vi "small_RT Main.vi"() -> ()   [LabVIEW 2018]
doc: "Demonstrates the use of the Network Streams functions to receive LED status from the host computer."
uses:
  <vilib>/myRIO/Instrument Drivers/Onboard IO/PWM/typedefs/PWM Reference.ctl
  <vilib>/myRIO/Common/Instrument Driver Framework/Utilities/typedefs/myRIO Generic Hardware Reference.ctl
  <vilib>/myRIO/Common/Instrument Driver Framework/Utilities/typedefs/Hardware Version Enum.ctl
  <vilib>/myRIO/Common/Instrument Driver Framework/Utilities/typedefs/myRIO v1.0 Reference.ctl
  <vilib>/myRIO/Common/Instrument Driver Framework/Utilities/typedefs/Generic FPGA Reference.ctl
  <vilib>/myRIO/Common/Instrument Driver Framework/myRIO v1.0/PWM/typedefs/PWM Channels Enum.ctl
  <vilib>/myRIO/Instrument Drivers/Onboard IO/PWM/typedefs/PWM Configuration.ctl
  <vilib>/userdefined/High Color/nirio_resource_hc.ctl
  <vilib>/myRIO/Instrument Drivers/Onboard IO/DIO/typedefs/DIO Reference.ctl
  <vilib>/myRIO/Common/Instrument Driver Framework/myRIO v1.0/DIO/typedefs/DIO Channels List.ctl
  <vilib>/myRIO/Common/Instrument Driver Framework/myRIO v1.0/DIO/typedefs/DIO Channels Enum.ctl
  <vilib>/myRIO/Common/Instrument Driver Framework/Utilities/vis/Is FPGA Ref Available.vi
  <vilib>/myRIO/Common/Instrument Driver Framework/myRIO v1.0/PWM/vis/myRIO v1.1 Open PWM.vi
  <vilib>/myRIO/Instrument Drivers/Onboard IO/PWM/vis/Set Duty Cycle and Frequency.vi
  <vilib>/myRIO/Common/Instrument Driver Framework/myRIO v1.0/DIO/vis/myRIO v1.1 Open DIO.vi
  <vilib>/myRIO/Instrument Drivers/Onboard IO/DIO/vis/Write.vi
  <vilib>/myRIO/Common/Instrument Driver Framework/Utilities/vis/Validate Channels.vi
  <vilib>/myRIO/Common/Instrument Driver Framework/myRIO v1.0/PWM/vis/myRIO v1.0 Reserve PWM.vi
  <vilib>/myRIO/Common/Instrument Driver Framework/myRIO v1.0/DIO/vis/myRIO v1.0 Reserve DIO.vi
  <vilib>/myRIO/Common/Instrument Driver Framework/myRIO v1.0/UART/vis/myRIO v1.0 Close UART.vi
  <vilib>/myRIO/Common/Instrument Driver Framework/myRIO v1.0/PWM/vis/myRIO v1.0 Build MUX Configuration PWM.vi
  <vilib>/myRIO/Common/Instrument Driver Framework/myRIO v1.0/Resource Manager/vis/myRIO v1.0 Reserve Channel List.vi
  <vilib>/myRIO/Common/Instrument Driver Framework/myRIO v1.0/DIO/vis/myRIO v1.0 Build MUX Configuration DIO.vi
  <vilib>/myRIO/Common/Instrument Driver Framework/myRIO v1.0/Resource Manager/vis/myRIO v1.0 Create Configuration List.vi
  <vilib>/myRIO/Common/Instrument Driver Framework/myRIO v1.0/Resource Manager/vis/myRIO v1.0 Reserve Channel.vi
  <vilib>/myRIO/Common/Instrument Driver Framework/myRIO v1.0/Resource Manager/vis/myRIO v1.0 Unreserve Channel.vi
  <vilib>/myRIO/Common/Instrument Driver Framework/myRIO v1.0/Resource Manager/vis/myRIO v1.0 Build Mutex Name.vi
  <vilib>/myRIO/Common/Instrument Driver Framework/Utilities/vis/FPGA Ref Manager.vi
  <vilib>/myRIO/Common/Instrument Driver Framework/myRIO v1.0/myRIO v1.0 Reset FPGA.vi
  <vilib>/myRIO/Common/Instrument Driver Framework/myRIO v1.0/IRQ/vis/myRIO v1.0 IRQ Info FGV.vi
  <vilib>/myRIO/Common/Instrument Driver Framework/myRIO v1.0/IRQ/vis/myRIO v1.0 Timer IRQ Info FGV.vi
  <vilib>/myRIO/Common/Instrument Driver Framework/myRIO v1.0/IRQ/vis/myRIO v1.0 ISR Agent.vi
  <vilib>/Utility/VariantDataType/GetNumericInfo.vi
  <vilib>/Utility/error.llb/Error Cluster From Error Code.vi
  <vilib>/myRIO/Common/Instrument Driver Framework/myRIO v1.0/myRIO v1.1 Open.vi
  <vilib>/myRIO/Common/Instrument Driver Framework/Utilities/vis/IO Manager.vi
  <vilib>/myRIO/Common/Instrument Driver Framework/Utilities/vis/Configuration Manager.vi
  <vilib>/myRIO/Common/Instrument Driver Framework/myRIO v1.0/Resource Manager/vis/myRIO v1.0 Configure IO.vi
  <vilib>/myRIO/Common/Instrument Driver Framework/myRIO v1.0/myRIO v1.0 Close.vi
  <vilib>/myRIO/Common/Instrument Driver Framework/myRIO v1.0/PWM/vis/myRIO v1.0 Write PWM.vi
  <vilib>/myRIO/Common/Instrument Driver Framework/myRIO v1.0/DIO/vis/myRIO v1.0 Write DIO.vi
  <vilib>/ErrorRing/Error Ring.xnode
  <vilib>/myRIO/Express VI/Onboard IO/PWM/PWM Express VI.xnode
  <vilib>/myRIO/Instrument Drivers/Onboard IO/PWM/vis/myRIO PWM Open.xnode
  <vilib>/myRIO/Express VI/Onboard IO/DO/DO Express VI.xnode
  <vilib>/myRIO/Instrument Drivers/Onboard IO/DIO/vis/myRIO DIO Open.xnode
  <vilib>/myRIO/Instrument Drivers/Utilities/Utilities.lvlib
  <vilib>/myRIO/Instrument Drivers/Onboard IO/PWM/PWM.lvlib
  <vilib>/myRIO/Instrument Drivers/Onboard IO/DIO/DIO.lvlib
panel:
  out "Stop_field":bool
  in  "l_gain":dbl=0.358
  in  "m_gain":dbl=0.353
  in  "s_gain":dbl=0.412
  in  "Enable":bool=TRUE
  in  "Frequency":dbl=1000.0
  out "L":dbl(graph)
  out "M":dbl(graph)
  out "S":dbl(graph)
  out "s":dbl format="%.3f"
  out "field error":errorcluster
  out "Receive":dbl[](array[numeric])
  out "loops":dbl
  out "error out":errorcluster
  in  "Stop":bool
  # "Overview: Demonstrates the use of the Network Streams functions to receive LED status from the host computer.\nInstructions:\n1. Run this VI.\n2. Open RT Main.vi and follow its front panel instructions.\n3. Click Stop to stop this VI. Stopping this VI also terminates the running of Desktop Main.vi."
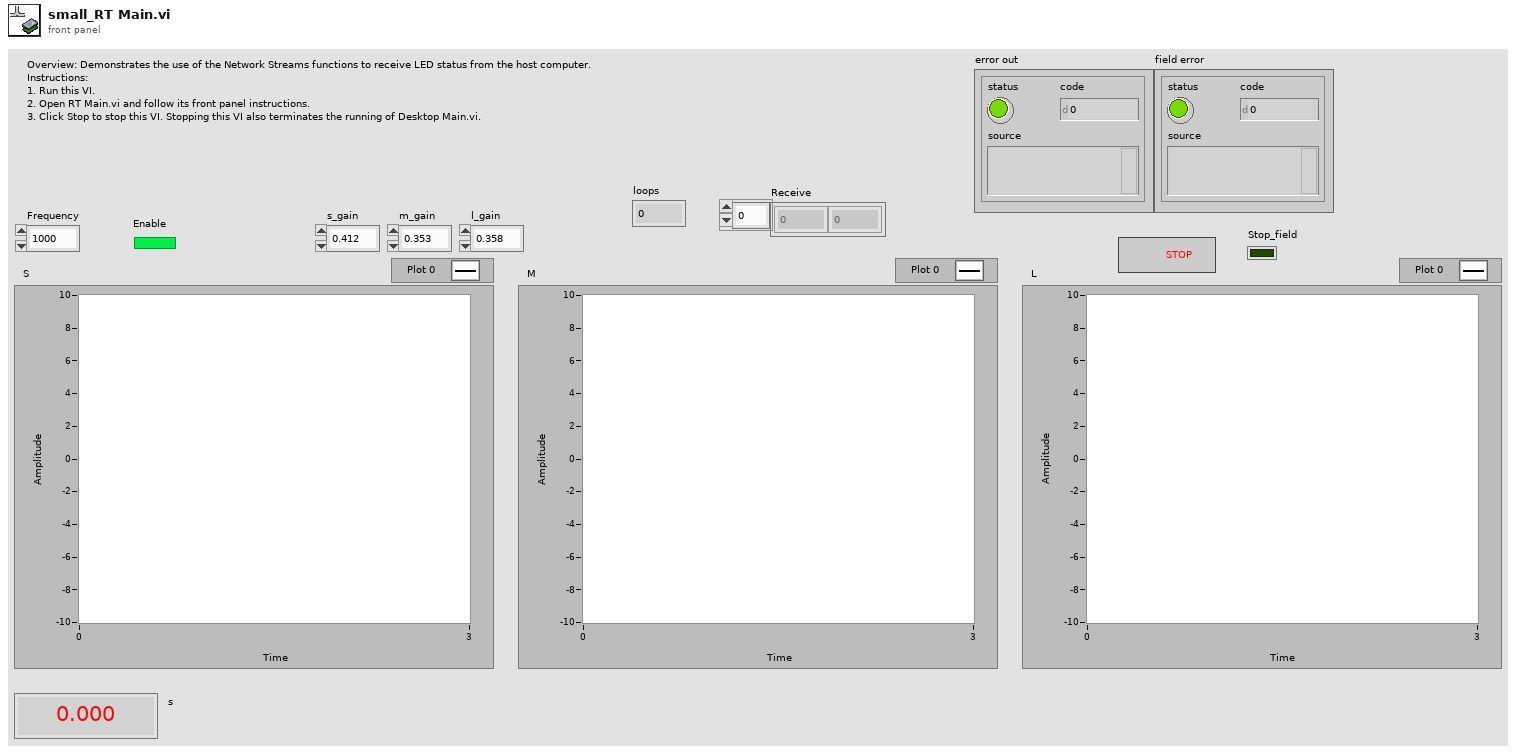
[diagram p1: front panel]
types:
  T1 = typedef "DIO.lvlib/DIO Reference.ctl" = cluster{"myRIO Reference":T2, "DIO Channels List":T6}
  T2 = typedef "myRIO Generic Hardware Reference.ctl" = cluster{"myRIO Model":T3, "myRIO Hardware Reference":T4}
  T3 = typedef "Hardware Version Enum.ctl" = enum16{"Unknown", "myRIO-1900", "myRIO-1950", "roboRIO", "NI ELVIS RIO CM", "ELVIS III"}
  T4 = typedef "myRIO v1.0 Reference.ctl" = cluster{"Generic FPGA Reference":T5, "Allow multiple opens":bool}
  T5 = typedef "Generic FPGA Reference.ctl" = refnum<k20>
  T6 = typedef "DIO Channels List.ctl" = T7[]
  T7 = typedef "DIO Channels Enum.ctl" = enum16{"Not Connected", "C/DIO0", "C/DIO1", "C/DIO2", "C/DIO3", "C/DIO4", "C/DIO5", "C/DIO6", "C/DIO7", "A/DIO0", "A/DIO1", "A/DIO2", "A/DIO3", "A/DIO4", "A/DIO5", "A/DIO6", "A/DIO7", "A/DIO8", "A/DIO9", "A/DIO10", "A/DIO11", "A/DIO12", "A/DIO13", "A/DIO14", "A/DIO15", "A/DIO16", "A/DIO17", "A/DIO18", "A/DIO19", "B/DIO0", "B/DIO1", "B/DIO2", "B/DIO3", "B/DIO4", "B/DIO5", "B/DIO6", "B/DIO7", "B/DIO8", "B/DIO9", "B/DIO10", "B/DIO11", "B/DIO12", "B/DIO13", "B/DIO14", "B/DIO15", "B/DIO16", "B/DIO17", "B/DIO18", "B/DIO19", "LED0", "LED1", "LED2", "LED3", "Button0", "DIO/DIO0", "DIO/DIO1", "DIO/DIO2", "DIO/DIO3", "DIO/DIO4", "DIO/DIO5", "DIO/DIO6", "DIO/DIO7", "DIO/DIO8", "DIO/DIO9", "SPI/CS0", "SPI/CS1", "SPI/CS2", "SPI/CS3", "LED RADIO (Green)", "LED RADIO (Red)", "LED COMM (Green)", "LED COMM (Red)", "LED MODE (Green)", "LED MODE (Red)"}
  T8 = typedef "nirio_resource_hc.ctl" = tag
  T9 = typedef "PWM.lvlib/PWM Reference.ctl" = cluster{"myRIO Reference":T2, "PWM Channels Enum":T10, "PWM Configuration":T11}
  T10 = typedef "PWM Channels Enum.ctl" = enum16{"Not Connected", "C/PWM0", "C/PWM1", "A/PWM0", "A/PWM1", "A/PWM2", "A/PWM3", "A/PWM4", "A/PWM5", "A/PWM6", "A/PWM7", "A/PWM8", "A/PWM9", "A/PWM10", "A/PWM11", "A/PWM12", "A/PWM13", "A/PWM14", "A/PWM15", "A/PWM16", "A/PWM17", "A/PWM18", "A/PWM19", "B/PWM0", "B/PWM1", "B/PWM2", "B/PWM3", "B/PWM4", "B/PWM5", "B/PWM6", "B/PWM7", "B/PWM8", "B/PWM9", "B/PWM10", "B/PWM11", "B/PWM12", "B/PWM13", "B/PWM14", "B/PWM15", "B/PWM16", "B/PWM17", "B/PWM18", "B/PWM19", "PWM/PWM0", "PWM/PWM1", "PWM/PWM2", "PWM/PWM3", "PWM/PWM4", "PWM/PWM5", "PWM/PWM6", "PWM/PWM7", "PWM/PWM8", "PWM/PWM9"}
  T11 = typedef "PWM.lvlib/PWM Configuration.ctl" = cluster{"Frequency":dbl, "Duty Cycle":dbl}
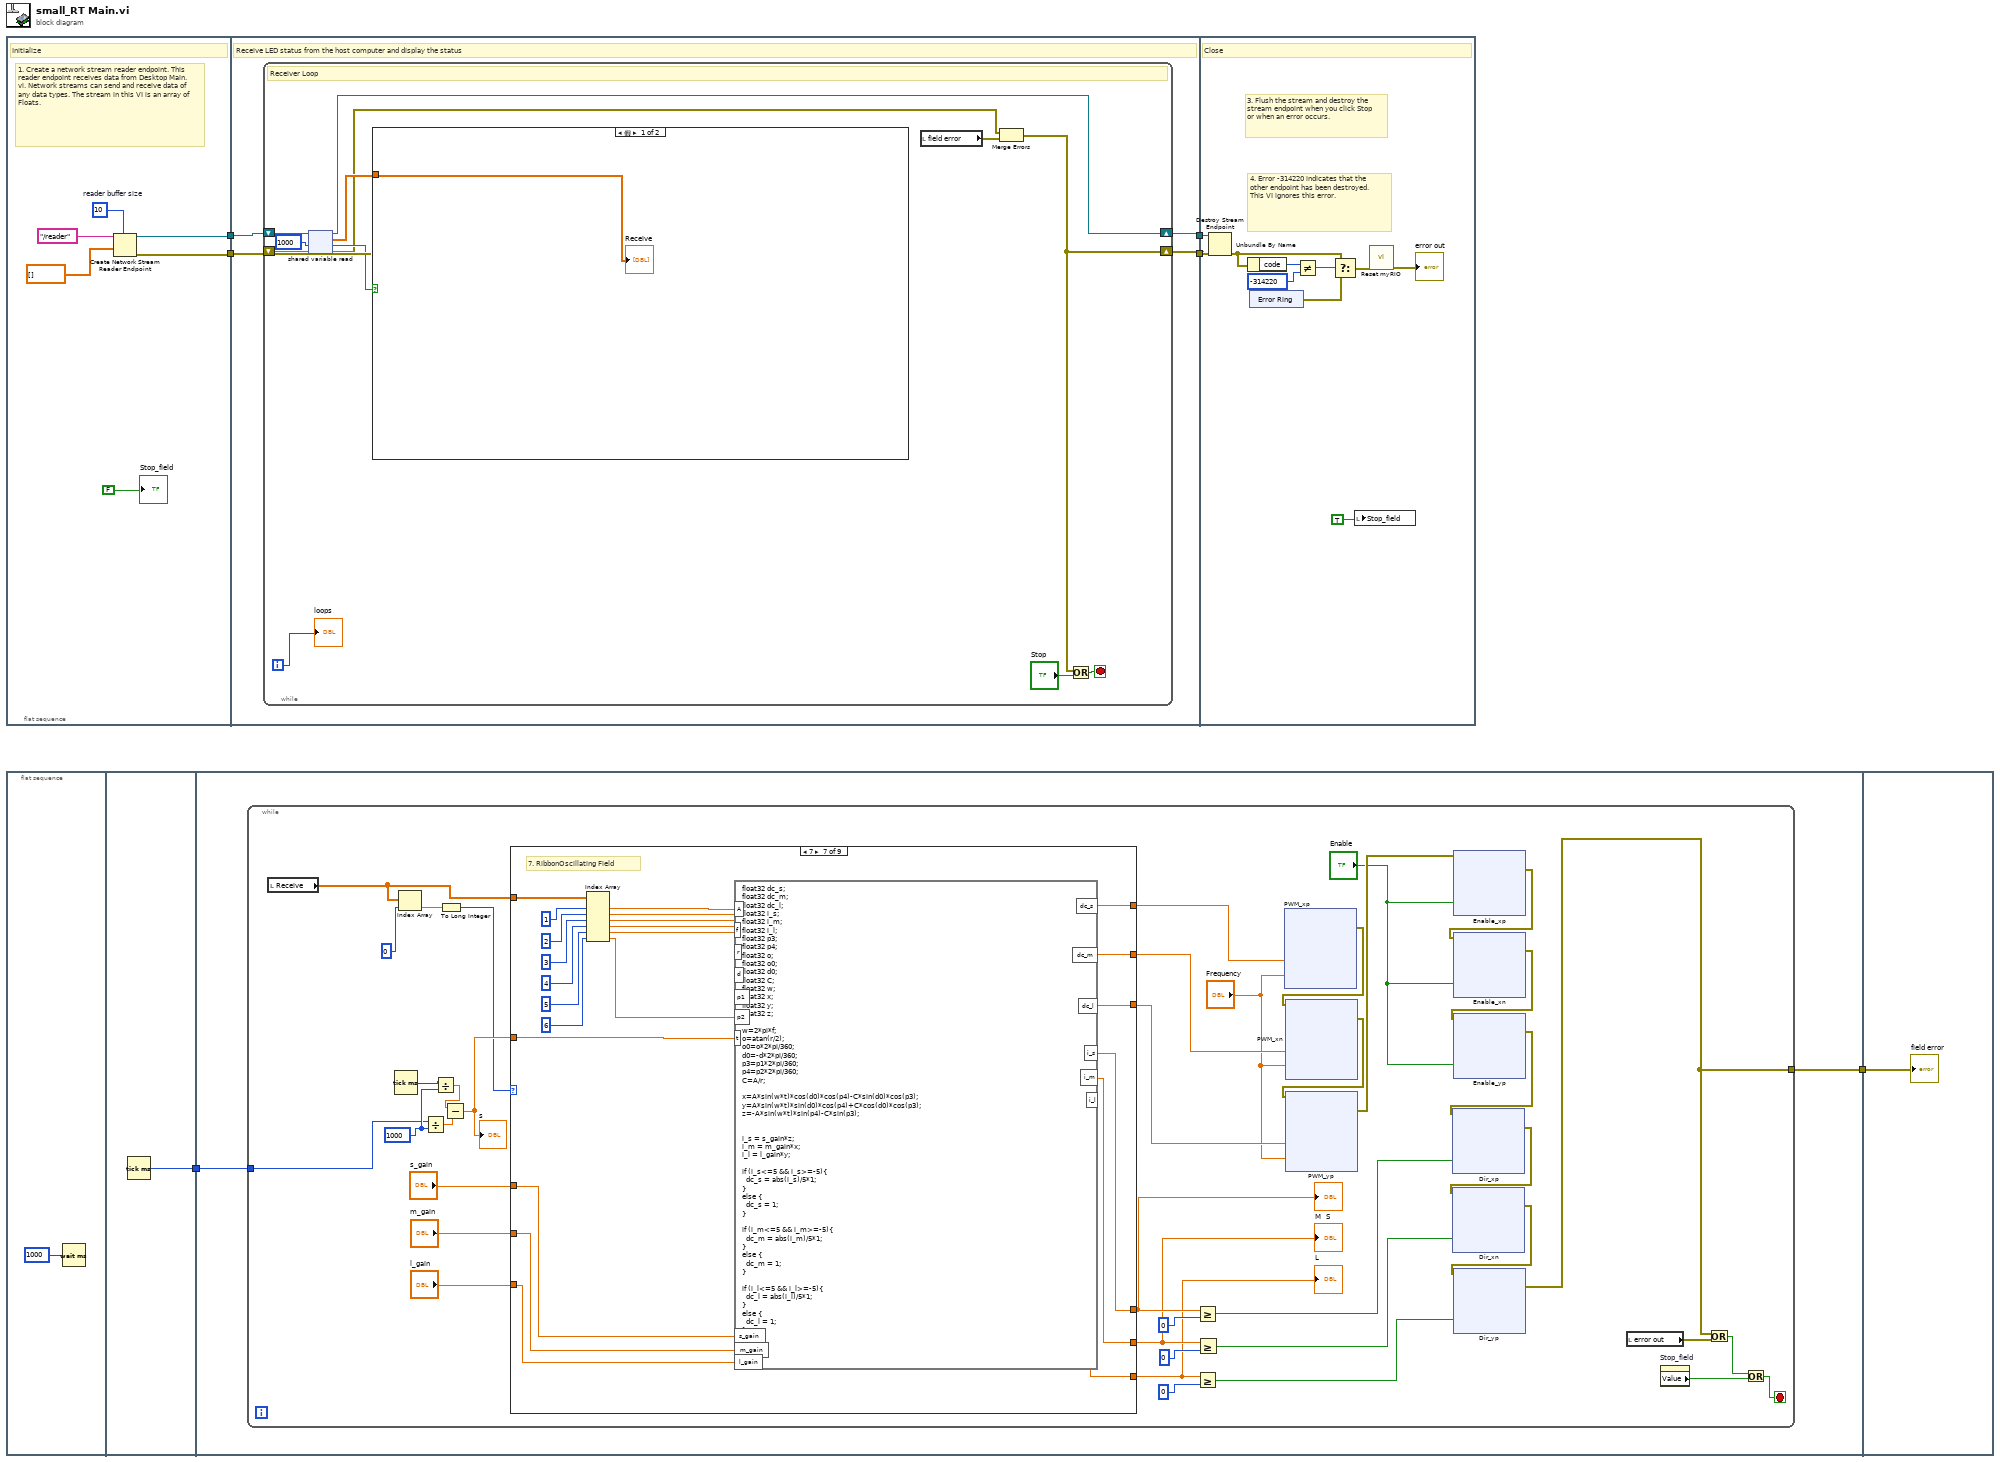
[diagram p0: block diagram]
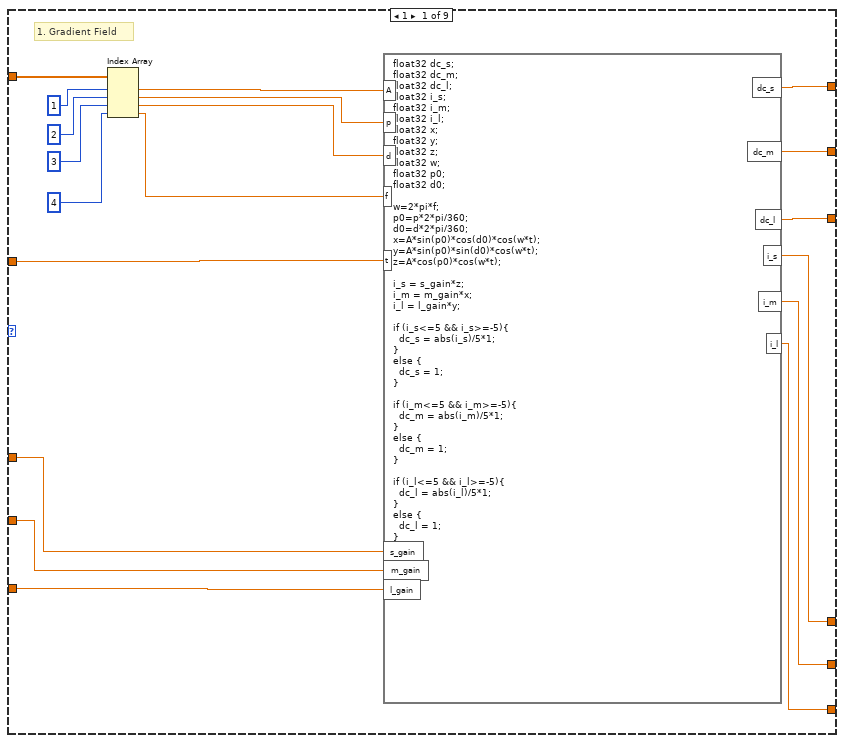
[diagram p2: hidden frame]
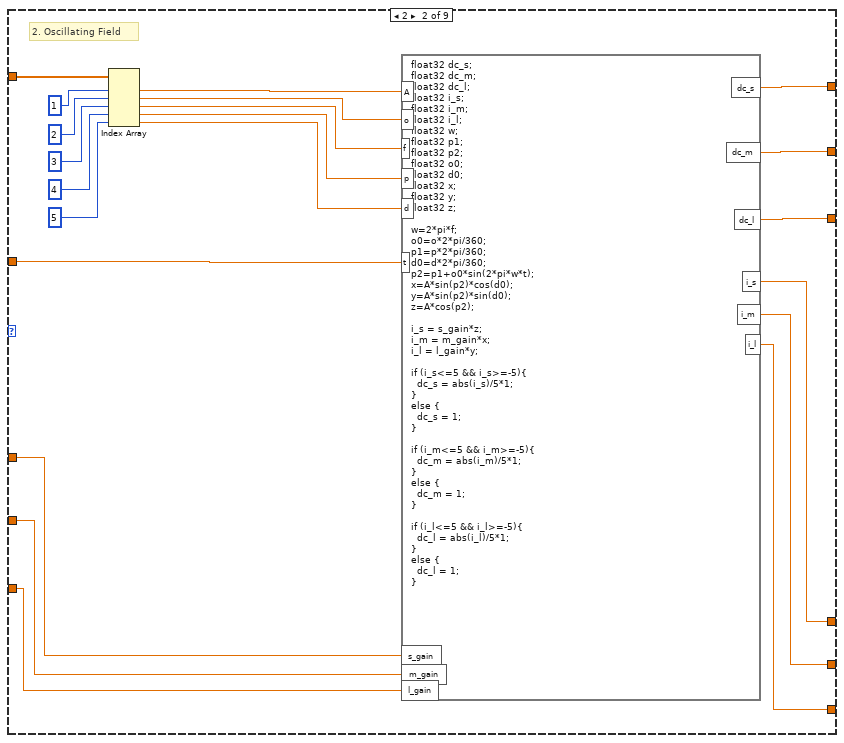
[diagram p3: hidden frame]
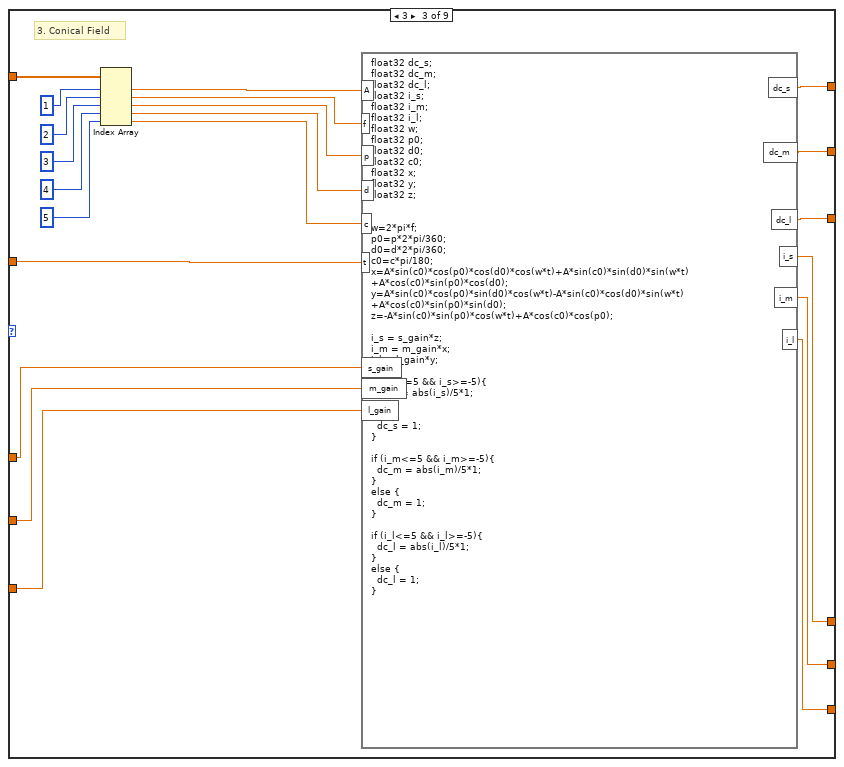
[diagram p4: hidden frame]
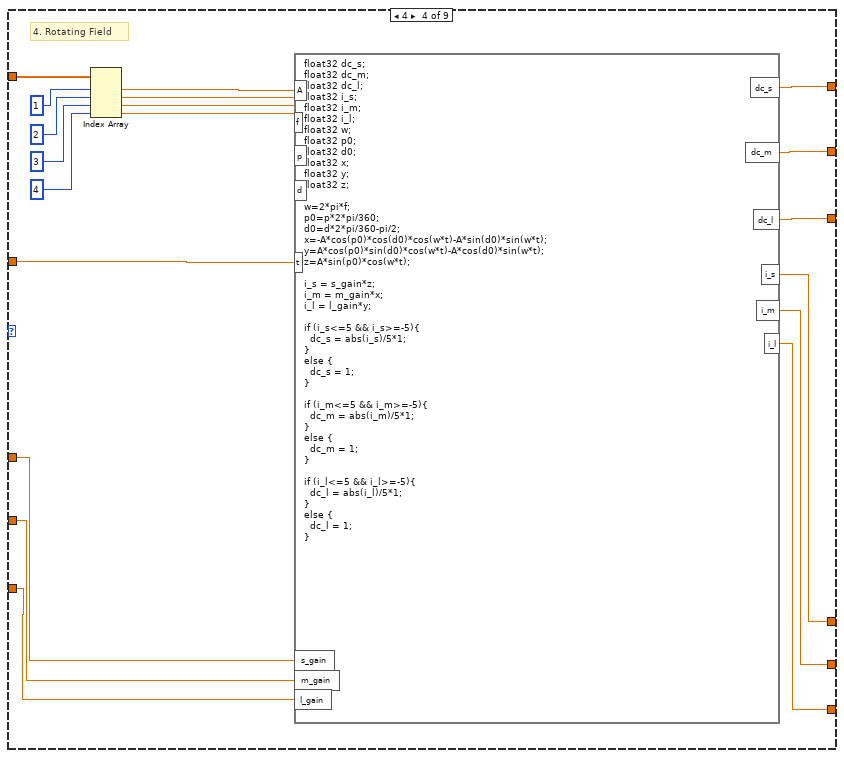
[diagram p5: hidden frame]
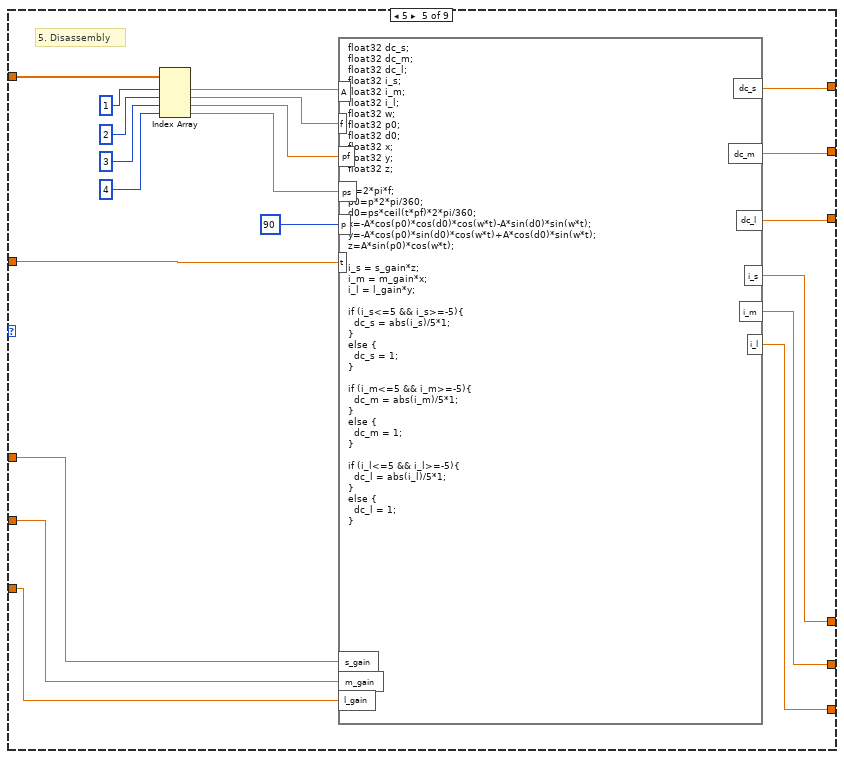
[diagram p6: hidden frame]
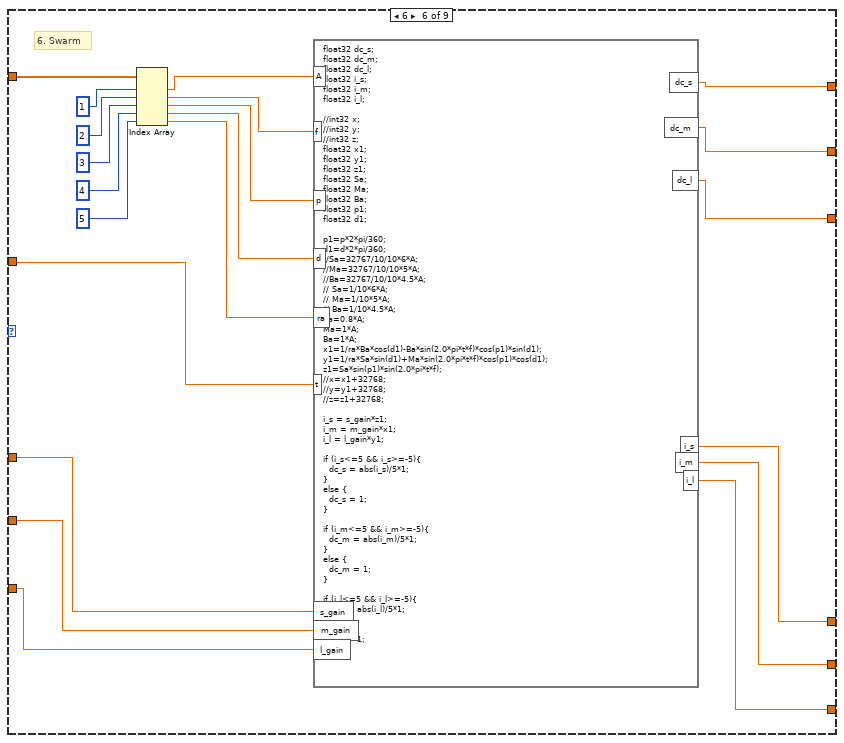
[diagram p7: hidden frame]
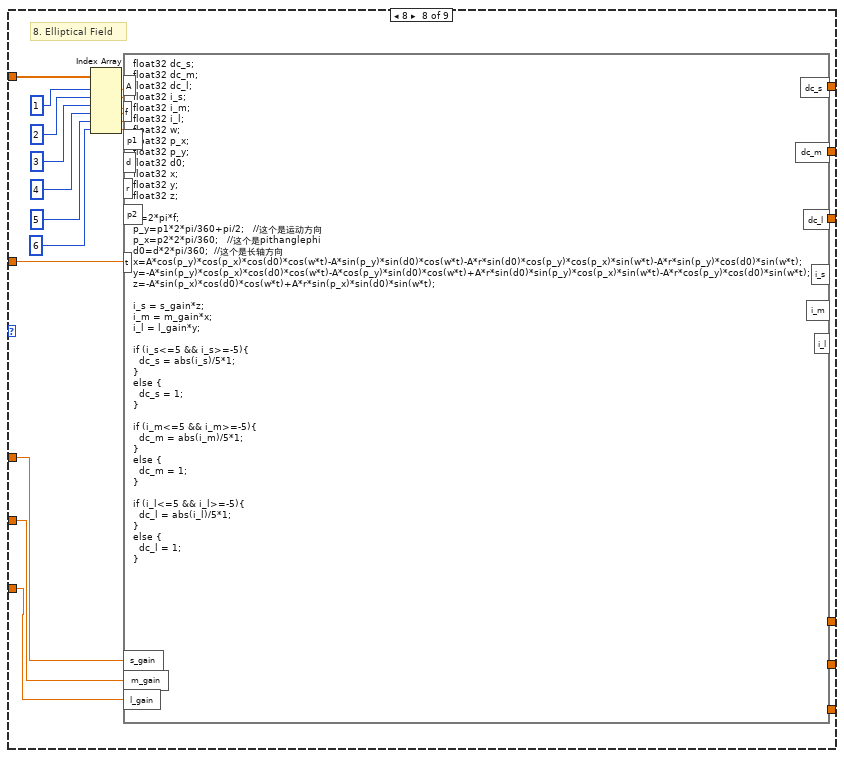
[diagram p8: hidden frame]
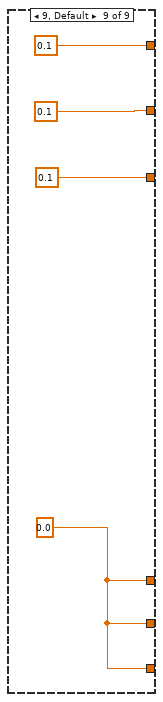
[diagram p9: hidden frame]
diagram:
  n1 = flat-sequence {
    tunnel: [w10] -> w3
    tunnel: [w9] -> w4
    tunnel: [w13] -> w6
    tunnel: [w14] -> w5
    tunnel: w3 -> [w16]
    tunnel: w4 -> [w15]
    tunnel: w6 -> [w39]
    tunnel: w5 -> [w38]
    frame #0 {
      w12 = 10  # reader buffer size
      # "1. Create a network stream reader endpoint. This reader endpoint receives data from Desktop Main.vi. Network streams can send and receive data of any data types. The stream in this VI is an array of Floats."
      # "Initialize"
      n2 = Create Network Stream Reader Endpoint(7:w12, 9:dbl[] [], 11:"/reader" ("reader name")) -> (0:w9:errorcluster, 3:w10:refnum<k21>)  [unwired: 4 in]
      "Stop_field" <- FALSE
    }
    frame #1 {
      # "Receive LED status from the host computer and display the status"
      n3 = while {
        shift-right: [w23] -> w13
        shift-left: w16 -> [w24]
        shift-right: [w18] -> w14
        shift-left: w15 -> [w26]
        i -> [w22]
        stop <- w27 stop-if-true
        # "Receiver Loop"
        n4 = shared-variable-read(w24, w26, 1000 ("timeout ms (-1)")) -> (w23:refnum<k21>, w17:errorcluster, w21:bool, w20:dbl[])
        n5 = case shown="假" w21 {
          tunnel: w20 -> [w29 _]
          frame False {
            "Receive" <- w29
          }
          frame True {
            # "time out occurs, no data is received"
          }
        }
        n6 = local read "field error"() -> (w19:errorcluster)
        n7 = Merge Errors(w17, w19) -> (w18:errorcluster)
        n8 = Or(x=w18, y="Stop") -> (x .or. y?=w27:bool)
        "loops" <- w22
      }
    }
    frame #2 {
      # "4. Error -314220 indicates that the other endpoint has been destroyed. This VI ignores this error."
      # "3. Flush the stream and destroy the stream endpoint when you click Stop or when an error occurs."
      # "Close"
      n9 = Destroy Stream Endpoint(8:w38, 11:w39) -> (0:w33:errorcluster)
      n10 = Unbundle By Name(w33) -> ("code"=w37:i32)
      n11 = xnode "Error Ring"() -> ("错误输出"=w34:errorcluster)
      n12 = Not Equal?(x=w37, y=-314220) -> (x != y?=w35:bool)
      n13 = Select(t=w33, s=w35, f=w34) -> (s? t:f=w32:errorcluster)
      n14 = local write "Stop_field"(TRUE) -> ()
      n15 = call <vilib>:"Reset myRIO.vi"("error in (no error)"=w32) -> ("error out"=→"error out":errorcluster)  [unwired: 10 in]
    }
  }
  n16 = flat-sequence {
    tunnel: [w42] -> w2
    tunnel: w2 -> [w44]
    tunnel: [w43] -> w1
    tunnel: w1 -> [w571]
    frame #0 {
      n17 = Wait (ms)(milliseconds to wait=1000) -> ()  [unwired: 1 out]
    }
    frame #1 {
      n18 = Tick Count (ms)() -> (millisecond timer value=w42:u32)
    }
    frame #2 {
      n19 = while {
        tunnel: w44 -> [w52]
        tunnel: [w51] -> w43
        stop <- w84 stop-if-true
        w81 = 1000
        n20 = local read "Receive"() -> (w53:dbl[])
        n21 = Tick Count (ms)() -> (millisecond timer value=w82:u32)
        n22 = Index Array(array=w53, index=0) -> (element=w77:dbl)
        n23 = Divide(x=w52, y=w81) -> (x/y=w83:dbl)
        n24 = Divide(x=w82, y=w81) -> (x/y=w80:dbl)
        n25 = To Long Integer(number=w77) -> (32bit integer=w76:i32)
        n26 = Subtract(x=w80, y=w83) -> (x-y=w78:dbl)
        "s" <- w78
        n27 = case shown="7" w76 {
          tunnel: w78 -> [w413 w433 w455 w479 w481 w510 w537 w566 _]
          tunnel: w53 -> [w414 w434 w456 w470 w495 w515 w538 w558 _]
          tunnel: [w410 w427 w448 w469 w494 w502 w531 w557 0.1] -> w75
          tunnel: [w409 w426 w447 w468 w493 w501 w530 w556 0.1] -> w74
          tunnel: [w408 w425 w446 w467 w492 w500 w529 w555 0.1] -> w73
          tunnel: [w407 w424 w445 w466 w491 w505 w528 w554 w567] -> w47
          tunnel: [w406 w423 w444 w465 w490 w504 w527 w553 w567] -> w46
          tunnel: [w405 w422 w443 w464 w489 w503 w526 w552 w567] -> w45
          tunnel: "s_gain" -> [w404 w421 w442 w463 w488 w508 w525 w551 _]
          tunnel: "m_gain" -> [w403 w420 w441 w462 w487 w507 w524 w550 _]
          tunnel: "l_gain" -> [w402 w419 w440 w461 w486 w506 w523 w549 _]
          frame 1 {
            # "1. Gradient Field"
            n28 = Index Array(array=w414, index #1=1, index #2=2, index #3=3, index #4=4) -> (element #1=w415:dbl, element #2=w412:dbl, element #3=w411:dbl, element #4=w400:dbl)
            n29 = formula code="float32 dc_s;\nfloat32 dc_m;\nfloat32 dc_l;\nfloat32 i_s;\nfloat32 i_m;\nfloat32 i_l;\nfloat32 x;\nfloat32 y;\nfloat32 z;\nfloat32 w;\nfloat32 p0;\nfloat32 d0;\n\nw=2*pi*f;\np0=p*2*pi/360;\nd0=d*2*pi/360;\nx=A*sin(p0)*cos(d0)*cos(w*t);\ny=A*sin(p0)*sin(d0)*cos(w*t);\nz=A*cos(p0)*cos(w*t);\n\ni_s = s_gain*z;\ni_m = m_gain*x;\ni_l = l_gain*y;\n\nif (i_s<=5 && i_s>=-5){\n  dc_s = abs(i_s)/5*1;\n}\nelse {\n  dc_s = 1;\n}\n\nif (i_m<=5 && i_m>=-5){\n  dc_m = abs(i_m)/5*1;\n}\nelse {\n  dc_m = 1;\n}\n\nif (i_l<=5 && i_l>=-5){\n  dc_l = abs(i_l)/5*1;\n}\nelse {\n  dc_l = 1;\n}"("t"=w413, "A"=w415, "p"=w412, "d"=w411, "s_gain"=w404, "m_gain"=w403, "l_gain"=w402, "f"=w400) -> ("dc_s"=w410:sgl, "dc_l"=w408:sgl, "i_s"=w407:sgl, "i_m"=w406:sgl, "i_l"=w405:sgl, "dc_m"=w409:sgl)
          }
          frame 2 {
            # "2. Oscillating Field"
            n30 = Index Array(array=w434, index #1=1, index #2=2, index #3=3, index #4=4, index #5=5) -> (element #1=w432:dbl, element #2=w431:dbl, element #3=w430:dbl, element #4=w429:dbl, element #5=w428:dbl)
            n31 = formula code="float32 dc_s;\nfloat32 dc_m;\nfloat32 dc_l;\nfloat32 i_s;\nfloat32 i_m;\nfloat32 i_l;\nfloat32 w;\nfloat32 p1;\nfloat32 p2;\nfloat32 o0;\nfloat32 d0;\nfloat32 x;\nfloat32 y;\nfloat32 z;\n\nw=2*pi*f;\no0=o*2*pi/360;\np1=p*2*pi/360;\nd0=d*2*pi/360;\np2=p1+o0*sin(2*pi*w*t);\nx=A*sin(p2)*cos(d0);\ny=A*sin(p2)*sin(d0);\nz=A*cos(p2);\n\ni_s = s_gain*z;\ni_m = m_gain*x;\ni_l = l_gain*y;\n\nif (i_s<=5 && i_s>=-5){\n  dc_s = abs(i_s)/5*1;\n}\nelse {\n  dc_s = 1;\n}\n\nif (i_m<=5 && i_m>=-5){\n  dc_m = abs(i_m)/5*1;\n}\nelse {\n  dc_m = 1;\n}\n\nif (i_l<=5 && i_l>=-5){\n  dc_l = abs(i_l)/5*1;\n}\nelse {\n  dc_l = 1;\n}"("t"=w433, "A"=w432, "f"=w430, "p"=w429, "d"=w428, "o"=w431, "s_gain"=w421, "m_gain"=w420, "l_gain"=w419) -> ("dc_s"=w427:sgl, "dc_l"=w425:sgl, "i_s"=w424:sgl, "i_m"=w423:sgl, "i_l"=w422:sgl, "dc_m"=w426:sgl)
          }
          frame 3 {
            # "3. Conical Field"
            n32 = Index Array(array=w456, index #1=1, index #2=2, index #3=3, index #4=4, index #5=5) -> (element #1=w454:dbl, element #2=w453:dbl, element #3=w452:dbl, element #4=w451:dbl, element #5=w449:dbl)
            n33 = formula code="float32 dc_s;\nfloat32 dc_m;\nfloat32 dc_l;\nfloat32 i_s;\nfloat32 i_m;\nfloat32 i_l;\nfloat32 w;\nfloat32 p0;\nfloat32 d0;\nfloat32 c0;\nfloat32 x;\nfloat32 y;\nfloat32 z;\n\n\nw=2*pi*f;\np0=p*2*pi/360;\nd0=d*2*pi/360;\nc0=c*pi/180;\nx=A*sin(c0)*cos(p0)*cos(d0)*cos(w*t)+A*sin(c0)*sin(d0)*sin(w*t)\n+A*cos(c0)*sin(p0)*cos(d0);\ny=A*sin(c0)*cos(p0)*sin(d0)*cos(w*t)-A*sin(c0)*cos(d0)*sin(w*t)\n+A*cos(c0)*sin(p0)*sin(d0);\nz=-A*sin(c0)*sin(p0)*cos(w*t)+A*cos(c0)*cos(p0);\n\ni_s = s_gain*z;\ni_m = m_gain*x;\ni_l = l_gain*y;\n\nif (i_s<=5 && i_s>=-5){\n  dc_s = abs(i_s)/5*1;\n}\nelse {\n  dc_s = 1;\n}\n\nif (i_m<=5 && i_m>=-5){\n  dc_m = abs(i_m)/5*1;\n}\nelse {\n  dc_m = 1;\n}\n\nif (i_l<=5 && i_l>=-5){\n  dc_l = abs(i_l)/5*1;\n}\nelse {\n  dc_l = 1;\n}"("t"=w455, "A"=w454, "f"=w453, "p"=w452, "d"=w451, "c"=w449, "s_gain"=w442, "m_gain"=w441, "l_gain"=w440) -> ("dc_s"=w448:sgl, "dc_l"=w446:sgl, "i_s"=w445:sgl, "i_m"=w444:sgl, "i_l"=w443:sgl, "dc_m"=w447:sgl)
          }
          frame 4 {
            # "4. Rotating Field"
            n34 = Index Array(array=w470, index #1=1, index #2=2, index #3=3, index #4=4) -> (element #1=w474:dbl, element #2=w473:dbl, element #3=w472:dbl, element #4=w471:dbl)
            n35 = formula code="float32 dc_s;\nfloat32 dc_m;\nfloat32 dc_l;\nfloat32 i_s;\nfloat32 i_m;\nfloat32 i_l;\nfloat32 w;\nfloat32 p0;\nfloat32 d0;\nfloat32 x;\nfloat32 y;\nfloat32 z;\n\nw=2*pi*f;\np0=p*2*pi/360;\nd0=d*2*pi/360-pi/2;\nx=-A*cos(p0)*cos(d0)*cos(w*t)-A*sin(d0)*sin(w*t);\ny=A*cos(p0)*sin(d0)*cos(w*t)-A*cos(d0)*sin(w*t);\nz=A*sin(p0)*cos(w*t);\n\ni_s = s_gain*z;\ni_m = m_gain*x;\ni_l = l_gain*y;\n\nif (i_s<=5 && i_s>=-5){\n  dc_s = abs(i_s)/5*1;\n}\nelse {\n  dc_s = 1;\n}\n\nif (i_m<=5 && i_m>=-5){\n  dc_m = abs(i_m)/5*1;\n}\nelse {\n  dc_m = 1;\n}\n\nif (i_l<=5 && i_l>=-5){\n  dc_l = abs(i_l)/5*1;\n}\nelse {\n  dc_l = 1;\n}"("t"=w479, "A"=w474, "f"=w473, "p"=w472, "d"=w471, "s_gain"=w463, "m_gain"=w462, "l_gain"=w461) -> ("dc_s"=w469:sgl, "dc_l"=w467:sgl, "i_s"=w466:sgl, "i_m"=w465:sgl, "i_l"=w464:sgl, "dc_m"=w468:sgl)
          }
          frame 5 {
            # "5. Disassembly"
            n36 = Index Array(array=w495, index #1=1, index #2=2, index #3=3, index #4=4) -> (element #1=w485:dbl, element #2=w484:dbl, element #3=w483:dbl, element #4=w482:dbl)
            n37 = formula code="float32 dc_s;\nfloat32 dc_m;\nfloat32 dc_l;\nfloat32 i_s;\nfloat32 i_m;\nfloat32 i_l;\nfloat32 w;\nfloat32 p0;\nfloat32 d0;\nfloat32 x;\nfloat32 y;\nfloat32 z;\n\nw=2*pi*f;\np0=p*2*pi/360;\nd0=ps*ceil(t*pf)*2*pi/360;\nx=-A*cos(p0)*cos(d0)*cos(w*t)-A*sin(d0)*sin(w*t);\ny=-A*cos(p0)*sin(d0)*cos(w*t)+A*cos(d0)*sin(w*t);\nz=A*sin(p0)*cos(w*t);\n\ni_s = s_gain*z;\ni_m = m_gain*x;\ni_l = l_gain*y;\n\nif (i_s<=5 && i_s>=-5){\n  dc_s = abs(i_s)/5*1;\n}\nelse {\n  dc_s = 1;\n}\n\nif (i_m<=5 && i_m>=-5){\n  dc_m = abs(i_m)/5*1;\n}\nelse {\n  dc_m = 1;\n}\n\nif (i_l<=5 && i_l>=-5){\n  dc_l = abs(i_l)/5*1;\n}\nelse {\n  dc_l = 1;\n}"("t"=w481, "A"=w485, "f"=w484, "pf"=w483, "ps"=w482, "s_gain"=w488, "m_gain"=w487, "l_gain"=w486, "p"=90) -> ("dc_s"=w494:sgl, "dc_l"=w492:sgl, "i_s"=w491:sgl, "i_m"=w490:sgl, "i_l"=w489:sgl, "dc_m"=w493:sgl)
          }
          frame 6 {
            # "6. Swarm"
            n38 = Index Array(array=w515, index #1=1, index #2=2, index #3=3, index #4=4, index #5=5) -> (element #1=w514:dbl, element #2=w513:dbl, element #3=w512:dbl, element #4=w511:dbl, element #5=w509:dbl)
            n39 = formula code="float32 dc_s;\nfloat32 dc_m;\nfloat32 dc_l;\nfloat32 i_s;\nfloat32 i_m;\nfloat32 i_l;\n\n//int32 x;\n//int32 y;\n//int32 z;\nfloat32 x1;\nfloat32 y1;\nfloat32 z1;\nfloat32 Sa;\nfloat32 Ma;\nfloat32 Ba;\nfloat32 p1;\nfloat32 d1;\n\np1=p*2*pi/360;\nd1=d*2*pi/360;\n//Sa=32767/10/10*6*A;\n//Ma=32767/10/10*5*A;\n//Ba=32767/10/10*4.5*A;\n// Sa=1/10*6*A;\n// Ma=1/10*5*A;\n// Ba=1/10*4.5*A;\nSa=0.8*A;\nMa=1*A;\nBa=1*A;\nx1=1/ra*Ba*cos(d1)-Ba*sin(2.0*pi*t*f)*cos(p1)*sin(d1);\ny1=1/ra*Sa*sin(d1)+Ma*sin(2.0*pi*t*f)*cos(p1)*cos(d1);\nz1=Sa*sin(p1)*sin(2.0*pi*t*f);\n//x=x1+32768;\n//y=y1+32768;\n//z=z1+32768;\n\ni_s = s_gain*z1;\ni_m = m_gain*x1;\ni_l = l_gain*y1;\n\nif (i_s<=5 && i_s>=-5){\n  dc_s = abs(i_s)/5*1;\n}\nelse {\n  dc_s = 1;\n}\n\nif (i_m<=5 && i_m>=-5){\n  dc_m = abs(i_m)/5*1;\n}\nelse {\n  dc_m = 1;\n}\n\nif (i_l<=5 && i_l>=-5){\n  dc_l = abs(i_l)/5*1;\n}\nelse {\n  dc_l = 1;\n}"("t"=w510, "A"=w514, "f"=w513, "p"=w512, "d"=w511, "ra"=w509, "s_gain"=w508, "m_gain"=w507, "l_gain"=w506) -> ("dc_s"=w502:sgl, "dc_m"=w501:sgl, "dc_l"=w500:sgl, "i_s"=w505:sgl, "i_m"=w504:sgl, "i_l"=w503:sgl)
          }
          frame 7 {
            # "7. RibbonOscillating Field"
            n40 = Index Array(array=w538, index #1=1, index #2=2, index #3=3, index #4=4, index #5=5, index #6=6) -> (element #1=w536:dbl, element #2=w535:dbl, element #3=w534:dbl, element #4=w533:dbl, element #5=w532:dbl, element #6=w521:dbl)
            n41 = formula code="float32 dc_s;\nfloat32 dc_m;\nfloat32 dc_l;\nfloat32 i_s;\nfloat32 i_m;\nfloat32 i_l;\nfloat32 p3;\nfloat32 p4;\nfloat32 o;\nfloat32 o0;\nfloat32 d0;\nfloat32 C;\nfloat32 w;\nfloat32 x;\nfloat32 y;\nfloat32 z;\n\nw=2*pi*f;\no=atan(r/2);\no0=o*2*pi/360;\nd0=-d*2*pi/360;\np3=p1*2*pi/360;\np4=p2*2*pi/360;\nC=A/r;\n\nx=A*sin(w*t)*cos(d0)*cos(p4)-C*sin(d0)*cos(p3);\ny=A*sin(w*t)*sin(d0)*cos(p4)+C*cos(d0)*cos(p3);\nz=-A*sin(w*t)*sin(p4)-C*sin(p3);\n\n\ni_s = s_gain*z;\ni_m = m_gain*x;\ni_l = l_gain*y;\n\nif (i_s<=5 && i_s>=-5){\n  dc_s = abs(i_s)/5*1;\n}\nelse {\n  dc_s = 1;\n}\n\nif (i_m<=5 && i_m>=-5){\n  dc_m = abs(i_m)/5*1;\n}\nelse {\n  dc_m = 1;\n}\n\nif (i_l<=5 && i_l>=-5){\n  dc_l = abs(i_l)/5*1;\n}\nelse {\n  dc_l = 1;\n}"("t"=w537, "A"=w536, "r"=w534, "d"=w533, "p1"=w532, "f"=w535, "s_gain"=w525, "m_gain"=w524, "l_gain"=w523, "p2"=w521) -> ("dc_s"=w531:sgl, "dc_l"=w529:sgl, "i_s"=w528:sgl, "i_m"=w527:sgl, "i_l"=w526:sgl, "dc_m"=w530:sgl)
          }
          frame 8 {
            # "8. Elliptical Field"
            n42 = Index Array ("索引数组")(array=w558, index #1=1, index #2=2, index #3=3, index #4=4, index #5=5, index #6=6) -> (element #1=w561:dbl, element #2=w560:dbl, element #3=w559:dbl, element #4=w546:dbl, element #5=w545:dbl, element #6=w544:dbl)
            n43 = formula code="float32 dc_s;\nfloat32 dc_m;\nfloat32 dc_l;\nfloat32 i_s;\nfloat32 i_m;\nfloat32 i_l;\nfloat32 w;\nfloat32 p_x;\nfloat32 p_y;\nfloat32 d0;\nfloat32 x;\nfloat32 y;\nfloat32 z;\n\nw=2*pi*f;\np_y=p1*2*pi/360+pi/2;   //这个是运动方向\np_x=p2*2*pi/360;   //这个是pithanglephi\nd0=d*2*pi/360;  //这个是长轴方向\nx=A*cos(p_y)*cos(p_x)*cos(d0)*cos(w*t)-A*sin(p_y)*sin(d0)*cos(w*t)-A*r*sin(d0)*cos(p_y)*cos(p_x)*sin(w*t)-A*r*sin(p_y)*cos(d0)*sin(w*t);      \ny=-A*sin(p_y)*cos(p_x)*cos(d0)*cos(w*t)-A*cos(p_y)*sin(d0)*cos(w*t)+A*r*sin(d0)*sin(p_y)*cos(p_x)*sin(w*t)-A*r*cos(p_y)*cos(d0)*sin(w*t);   \nz=-A*sin(p_x)*cos(d0)*cos(w*t)+A*r*sin(p_x)*sin(d0)*sin(w*t);\n\ni_s = s_gain*z;\ni_m = m_gain*x;\ni_l = l_gain*y;\n\nif (i_s<=5 && i_s>=-5){\n  dc_s = abs(i_s)/5*1;\n}\nelse {\n  dc_s = 1;\n}\n\nif (i_m<=5 && i_m>=-5){\n  dc_m = abs(i_m)/5*1;\n}\nelse {\n  dc_m = 1;\n}\n\nif (i_l<=5 && i_l>=-5){\n  dc_l = abs(i_l)/5*1;\n}\nelse {\n  dc_l = 1;\n}"("t"=w566, "A"=w561, "f"=w560, "p1"=w559, "d"=w546, "s_gain"=w551, "m_gain"=w550, "l_gain"=w549, "r"=w545, "p2"=w544) -> ("dc_s"=w557:sgl, "dc_l"=w555:sgl, "i_s"=w554:sgl, "i_m"=w553:sgl, "i_l"=w552:sgl, "dc_m"=w556:sgl)
          }
          frame 9, Default {
            w567 = 0.0
          }
        }
        "S" <- w47
        "M" <- w46
        "L" <- w45
        n44 = Greater Or Equal?(x=w47, y=0) -> (x >= y?=w68:bool)
        n45 = Greater Or Equal?(x=w45, y=0) -> (x >= y?=w64:bool)
        n46 = Greater Or Equal?(x=w46, y=0) -> (x >= y?=w65:bool)
        n47 = xnode "PWM_xp"("Duty Cycle"=w75, "Frequency [Hz]"="Frequency") -> ("error out"=w71:errorcluster)  [unwired: 1 in]
        n48 = xnode "PWM_xn"("Duty Cycle"=w74, "Frequency [Hz]"="Frequency", "error in (no error)"=w71) -> ("error out"=w70:errorcluster)
        n49 = xnode "PWM_yp"("Duty Cycle"=w73, "Frequency [Hz]"="Frequency", "error in (no error)"=w70) -> ("error out"=w62:errorcluster)
        n50 = xnode "Enable_xp"("A/DIO1 (Pin 13)"="Enable", "error in (no error)"=w62) -> ("error out"=w63:errorcluster)
        n51 = xnode "Enable_xn"("A/DIO3 (Pin 17)"="Enable", "error in (no error)"=w63) -> ("error out"=w61:errorcluster)
        n52 = xnode "Enable_yp"("A/DIO5 (Pin 21)"="Enable", "error in (no error)"=w61) -> ("error out"=w60:errorcluster)
        n53 = xnode "Dir_xp"("A/DIO0 (Pin 11)"=w68, "error in (no error)"=w60) -> ("error out"=w59:errorcluster)
        n54 = xnode "Dir_xn"("A/DIO2 (Pin 15)"=w65, "error in (no error)"=w59) -> ("error out"=w58:errorcluster)
        n55 = xnode "Dir_yp"("A/DIO4 (Pin 19)"=w64, "error in (no error)"=w58) -> ("error out"=w51:errorcluster)
        n56 = local read "error out"() -> (w50:errorcluster)
        n57 = property on="Stop_field" class="Bool (严格)"() -> ("Value"=w48:bool)  [unwired: 2 in, 2 out]
        n58 = Or(x=w51, y=w50) -> (x .or. y?=w49:bool)
        n59 = Or(x=w49, y=w48) -> (x .or. y?=w84:bool)
      }
    }
    frame #3 {
      "field error" <- w571
    }
  }
